vi "pc_convstring.vi"(1 "trimmed string":string) -> (0 "number":i32)   [LabVIEW 2009]
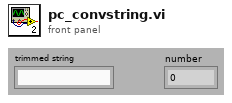
[diagram p1: front panel]
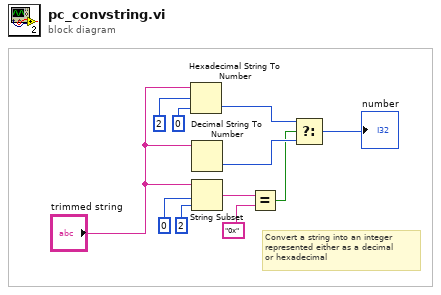
[diagram p0: block diagram]
diagram:
  # "Convert a string into an integer\nrepresented either as a decimal \nor hexadecimal"
  n1 = Hexadecimal String To Number(string="trimmed string", offset=2 ("Offset"), default (0uL)=0 ("Standard (0 U32)")) -> (number=w8:i32)  [unwired: 1 out]
  n2 = Decimal String To Number(string="trimmed string") -> (number=w6:i32)  [unwired: 2 in, 1 out]
  n3 = String Subset(string="trimmed string", offset (0)=0 ("Offset (0)"), length (rest)=2 ("Länge (Rest)")) -> (substring=w3:string)
  n4 = Equal?(x=w3, y="0x") -> (x = y?=w5:bool)
  n5 = Select(t=w8, s=w5, f=w6) -> (s? t:f=→"number":i32)
